vi "OpenPump.vi"(7 "ValidCh":T1[](array[typedef]) items=["7"=7, "11"=11, "12"=12, "13"=13, "15"=15, "16"=16, "18"=18, "29"=29, "32"=32, "33"=33, "35"=35, "36"=36, "37"=37, "38"=38, "40"=40], 8 "error in":errorcluster, 9 "Channel No in":T1=29 items=["7"=7, "11"=11, "12"=12, "13"=13, "15"=15, "16"=16, "18"=18, "29"=29, "32"=32, "33"=33, "35"=35, "36"=36, "37"=37, "38"=38, "40"=40], 10 "PI_REF":T3, 11 "CHStIn":T2) -> (0 "error out":errorcluster, 2 "Channel No out":T1 items=["7"=7, "11"=11, "12"=12, "13"=13, "15"=15, "16"=16, "18"=18, "29"=29, "32"=32, "33"=33, "35"=35, "36"=36, "37"=37, "38"=38, "40"=40], 3 "Output Value":bool)   [LabVIEW 2021, in "ValveCTRL.lvlib"]
uses:
  ValveCTRL.lvlib
  TypeDef/CHs_List.ctl
  <vilib>/MakerHub/LINX/Private/Type Defs/LINX Ref.ctl
  <vilib>/MakerHub/LINX/Private/Type Defs/Platform.ctl
  <vilib>/MakerHub/LINX/Private/Type Defs/Interface.ctl
  <vilib>/MakerHub/LINX/Private/Device/Type Defs/LINX Device Config.ctl
  <vilib>/MakerHub/LINX/Private/Device/Type Defs/TCP Config.ctl
  <vilib>/MakerHub/LINX/Private/Device/Type Defs/Channels.ctl
  TypeDef/ChannelStatus.ctl
  <vilib>/ErrorRing/Error Ring.xnode
  Main/Main.lvlib
  <vilib>/MakerHub/LINX/LMH-LINX.lvlib
  <vilib>/MakerHub/LINX/Private/Device/Device.lvlib
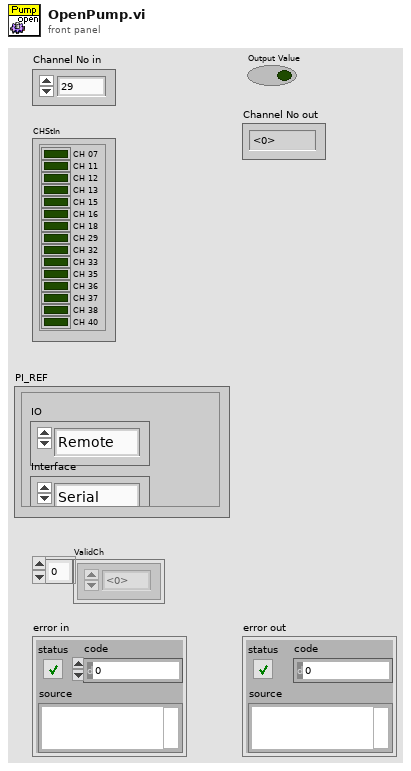
[diagram p1: front panel]
types:
  T1 = typedef "ValveCTRL.lvlib/CHs_List.ctl" = u8
  T2 = typedef "ValveCTRL.lvlib/ChannelStatus.ctl" = cluster{"CH 07":bool, "CH 11":bool, "CH 12":bool, "CH 13":bool, "CH 15":bool, "CH 16":bool, "CH 18":bool, "CH 29":bool, "CH 32":bool, "CH 33":bool, "CH 35":bool, "CH 36":bool, "CH 37":bool, "CH 38":bool, "CH 40":bool}
  T3 = typedef "LMH-LINX.lvlib/LINX Ref.ctl" = cluster{"IO":T4, "Interface":T5, "LINX Device Config":T6}
  T4 = typedef "LMH-LINX.lvlib/Platform.ctl" = enum16{"Remote", "Local"}
  T5 = typedef "LMH-LINX.lvlib/Interface.ctl" = enum16{"Serial", "TCP"}
  T6 = typedef "LMH-LINX.lvlib/Device.lvlib/LINX Device Config.ctl" = cluster{"Interface":T5, "COM Port":refnum<visa-resource-name>, "TCP Configuration":T7, "Device Family":u8, "Device ID":u8, "Device Name":string, "TCP Ref":refnum<k5>, "Channels":T8}
  T7 = typedef "LMH-LINX.lvlib/Device.lvlib/TCP Config.ctl" = cluster{"IP Address":string, "Port":u16}
  T8 = typedef "LMH-LINX.lvlib/Channels.ctl" = cluster{"DI":u8[], "DO":u8[], "AI":u8[], "AO":u8[], "PWM":u8[], "QE":u8[], "UART":u8[], "I2C 2":u8[], "SPI":u8[], "CAN":u8[], "Servo":u8[], "AI Ref (V)":dbl, "AI Resolution (Bits)":u8, "AO Ref (V)":dbl, "AO Resolution (Bits)":u8}
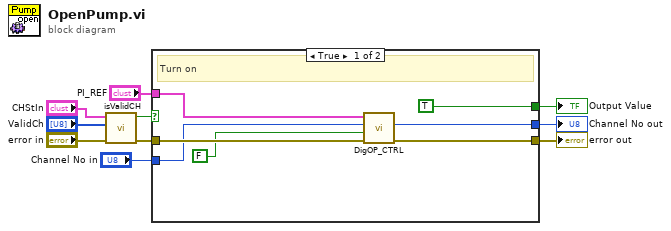
[diagram p0: block diagram]
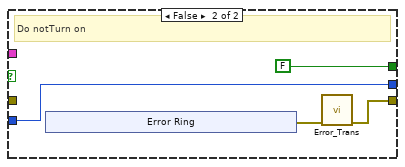
[diagram p2: hidden frame]
diagram:
  n1 = call "isValidCH.vi"("error in"="error in", "ValidCh"="ValidCh", "CHStIn"="CHStIn") -> ("error out"=w4:errorcluster, "VaildCH?"=w3:bool)  [unwired: 7 in]
  n2 = case shown="True" w3 {
    tunnel: [w16 w18] -> w8
    tunnel: w4 -> [w17 _]
    tunnel: [w14 w20] -> w5
    tunnel: [TRUE ("Output Value") FALSE ("Output Value")] -> w6
    tunnel: "Channel No in" -> [w12 w20]
    tunnel: "PI_REF" -> [w11 _]
    frame True {
      # "Turn on"
      n3 = call "DigOP_CTRL.vi"("Error In"=w17, "Output Value"=FALSE, "Channel No"=w12, "LINX Resource In"=w11) -> ("Error Out"=w16:errorcluster, "Channel No"=w14:T1)  [unwired: 5 in, 1 out]
    }
    frame False {
      # "Do notTurn on"
      n4 = xnode "Error Ring"() -> ("error out"=w19:errorcluster)
      n5 = call "Error_Trans.vi"("Error In"=w19) -> ("Error Out"=w18:errorcluster)  [unwired: 9 in, 1 out]
    }
  }
  "error out" <- w8
  "Output Value" <- w6
  "Channel No out" <- w5
